vi "Draw Text (Greyscale).vi"(4 "Text Drawing Settings (Default: Simplex)":T1={"OpenCV Font Face"=enum."FONT_HERSHEY_SIMPLEX", "Font Scale"=1.0}, 5 "Thickness (Default: 1)":i32=1, 6 "OpenCV Line Type (Default LINE_8)":T5=enum."LINE_8", 7 "Colour":u8=255, 8 "error in (no error)":errorcluster, 9 "Text":string, 10 "Origin":T3, 11 "Greyscale Image in":T4) -> (0 "error out":errorcluster, 3 "Greyscale Image":T4)   [LabVIEW 2020, in "image.lvlib"]
doc: "Draw the specified text with the given parameters.\n\nUse \"Get Text Size.vi\" if the size of the drawn-text needs to be determined for positioning purposes and use \"Required Font-Scale.vi\" to calculate a suitable font-scale to match the desired Text Height."
uses:
  image.lvlib
  Line Type.ctl
  Greyscale Image.ctl
  common/Image Point (Integer).ctl
  Text Drawing Settings.ctl
  Font Face.ctl
  0015c4fc-6a12-4f82-815b-6c2f827f408b.vi
  <vilib>/Utility/error.llb/Error Cluster From Error Code.vi
  common/common.lvlib
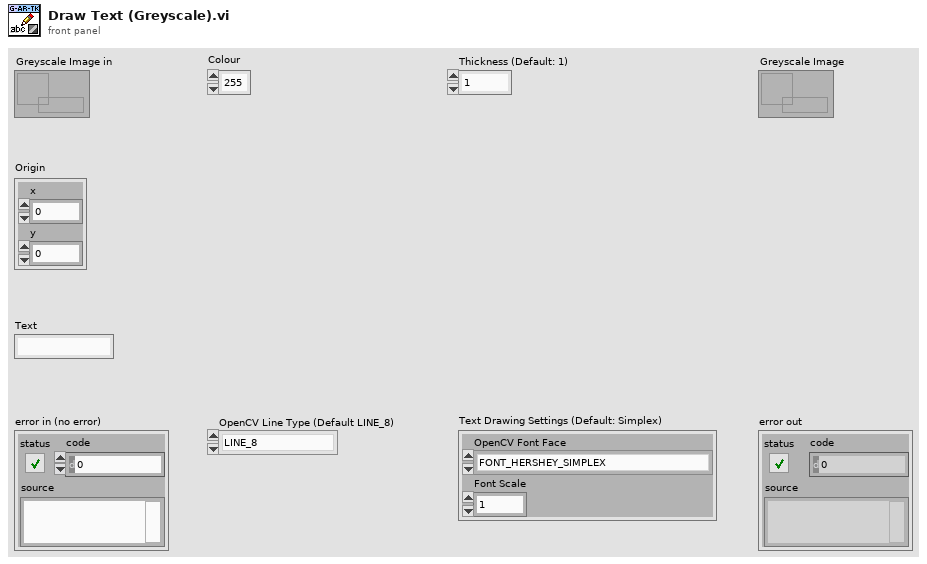
[diagram p1: front panel]
types:
  T1 = typedef "image.lvlib/Text Drawing Settings.ctl" = cluster{"OpenCV Font Face":T2, "Font Scale":dbl}
  T2 = typedef "image.lvlib/Font Face.ctl" = enum8{"FONT_HERSHEY_SIMPLEX", "FONT_HERSHEY_PLAIN", "FONT_HERSHEY_DUPLEX", "FONT_HERSHEY_COMPLEX", "FONT_HERSHEY_TRIPLEX", "FONT_HERSHEY_COMPLEX_SMALL", "FONT_HERSHEY_SCRIPT_SIMPLEX", "FONT_HERSHEY_SCRIPT_COMPLEX", "FONT_ITALIC"}
  T3 = typedef "common.lvlib/Image Point (Integer).ctl" = cluster{"x":i32, "y":i32}
  T4 = typedef "image.lvlib/Greyscale Image.ctl" = refnum<data-value>
  T5 = typedef "image.lvlib/Line Type.ctl" = enum8{"FILLED", "LINE_4", "LINE_8", "LINE_AA"}
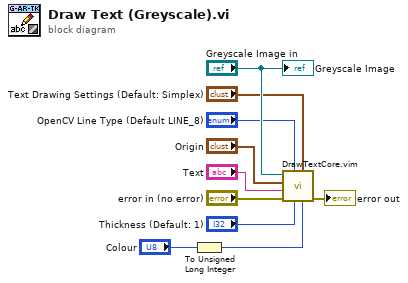
[diagram p0: block diagram]
diagram:
  n1 = To Unsigned Long Integer(number="Colour") -> (unsigned 32bit integer=w1:u32)
  n2 = call "DrawTextCore.vim"("Colour"=w1, "Text Drawing Settings"="Text Drawing Settings (Default: Simplex)", "Thickness"="Thickness (Default: 1)", "OpenCV Line Type"="OpenCV Line Type (Default LINE_8)", "error in (no error)"="error in (no error)", "Text"="Text", "Origin"="Origin", "Src"="Greyscale Image in") -> ("error out"=→"error out":errorcluster)  [unwired: 3 in]
  "Greyscale Image" <- "Greyscale Image in"
